vi "Write 2D Array.vi"(8 "error in (no error)":errorcluster, 10 "2D Array":dbl[][](array[numeric]), 11 "Data2D in":refnum<class "Data2D.lvclass">) -> (0 "error out":errorcluster, 3 "Data2D out":refnum<class "Data2D.lvclass">)   [LabVIEW 2014, in "Data2D.lvclass"]
uses:
  Data2D.lvclass
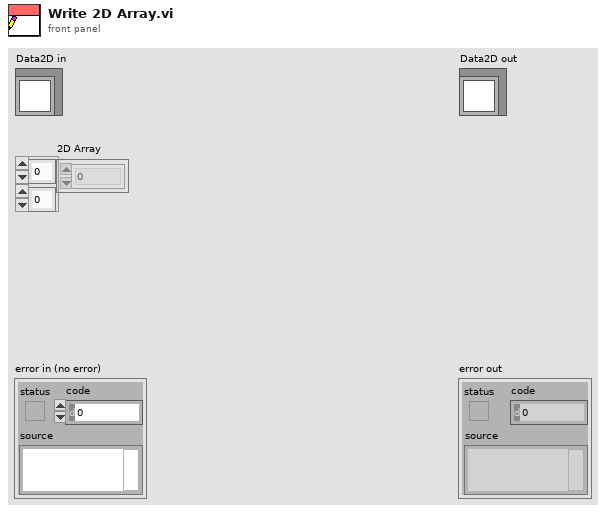
[diagram p1: front panel]
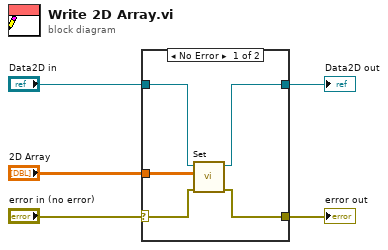
[diagram p0: block diagram]
diagram:
  n1 = case shown="No Error" "error in (no error)" {
    selector: "error in (no error)" -> [w7 w11]
    tunnel: [w6 w11] -> w4
    tunnel: [w8 w12] -> w2
    tunnel: "Data2D in" -> [w9 w12]
    tunnel: "2D Array" -> [w10 _]
    frame No Error {
      n2 = call-dynamic "Set.vi"("error in (no error)"=w7, "Data"=w10, "AbstractData in"=w9) -> ("error out"=w6:errorcluster, "AbstractData out"=w8:refnum<class "Data2D.lvclass">)  [unwired: 7 in]
    }
    frame Error {
    }
  }
  "error out" <- w4
  "Data2D out" <- w2
